vi "Get Top and Bottom Three.vi"(10 "Name Array":string[](array[string]), 11 "Stat Array":dbl[](array[numeric])) -> (3 "Top and Bottom 3":T1)   [LabVIEW 2020]
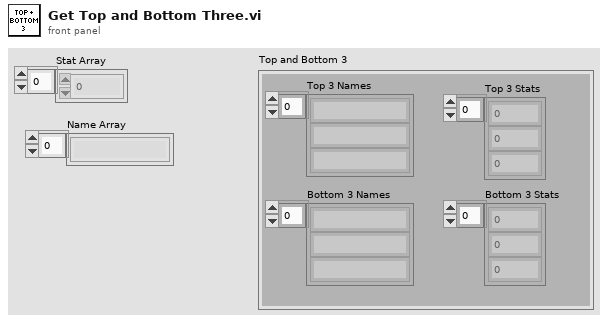
[diagram p1: front panel]
types:
  T1 = cluster{"Top 3 Names":string[], "Top 3 Stats":dbl[], "Bottom 3 Names":string[], "Bottom 3 Stats":dbl[]}
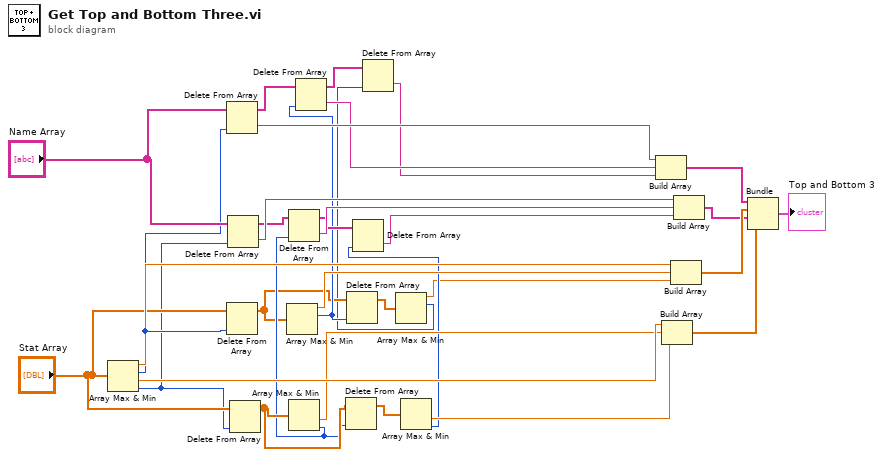
[diagram p0: block diagram]
diagram:
  n1 = Array Max & Min(array="Stat Array") -> (max value=w33:dbl, max index (indices)=w29:i32, min value=w32:dbl, min index (indices)=w28:i32)
  n2 = Delete From Array(array="Name Array", index=w29) -> (deleted portion=w26:string, array with subset deleted=w24:string[])  [unwired: 1 in]
  n3 = Delete From Array(array="Stat Array", index=w29) -> (array with subset deleted=w11:dbl[])  [unwired: 1 in, 1 out]
  n4 = Delete From Array(array="Name Array", index=w28) -> (deleted portion=w25:string, array with subset deleted=w21:string[])  [unwired: 1 in]
  n5 = Delete From Array(array="Stat Array", index=w28) -> (array with subset deleted=w19:dbl[])  [unwired: 1 in, 1 out]
  n6 = Array Max & Min(array=w11) -> (max value=w27:dbl, max index (indices)=w12:i32)  [unwired: 2 out]
  n7 = Array Max & Min(array=w19) -> (min value=w22:dbl, min index (indices)=w18:i32)  [unwired: 2 out]
  n8 = Delete From Array(array=w21, index=w18) -> (deleted portion=w20:string, array with subset deleted=w15:string[])  [unwired: 1 in]
  n9 = Delete From Array(array=w24, index=w12) -> (deleted portion=w23:string, array with subset deleted=w7:string[])  [unwired: 1 in]
  n10 = Delete From Array(array=w19, index=w18) -> (array with subset deleted=w17:dbl[])  [unwired: 1 in, 1 out]
  n11 = Delete From Array(array=w11, index=w12) -> (array with subset deleted=w9:dbl[])  [unwired: 1 in, 1 out]
  n12 = Array Max & Min(array=w9) -> (max value=w10:dbl, max index (indices)=w8:i32)  [unwired: 2 out]
  n13 = Delete From Array(array=w7, index=w8) -> (deleted portion=w6:string)  [unwired: 1 in, 1 out]
  n14 = Array Max & Min(array=w17) -> (min value=w16:dbl, min index (indices)=w14:i32)  [unwired: 2 out]
  n15 = Delete From Array(array=w15, index=w14) -> (deleted portion=w13:string)  [unwired: 1 in, 1 out]
  n16 = Build Array(w26, w23, w6) -> (w5:string[])
  n17 = Build Array(w32, w22, w16) -> (w2:dbl[])
  n18 = Build Array(w33, w27, w10) -> (w4:dbl[])
  n19 = Build Array(w25, w20, w13) -> (w3:string[])
  n20 = Bundle(w5, w4, w3, w2) -> (→"Top and Bottom 3":cluster{string[], dbl[], string[], dbl[]})  [unwired: 1 in]
